vi "resetHomePosition.vi"(8 "error in (no error)":errorcluster, 11 "VISA Refnum in":refnum<visa-resource-name>) -> (0 "error out":errorcluster, 3 "VISA Refnum out":refnum<visa-resource-name>)   [LabVIEW 2014]
doc: "Newport Motion Controler\nThis VI reset HOME position\n\nAndré Romero - 2020\nandretec@ifsc.usp.br"
uses:
  <userlib>/Newport ESP301/Newport ESP301.lvlib
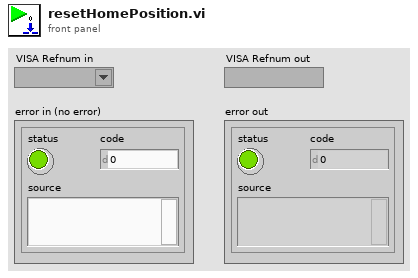
[diagram p1: front panel]
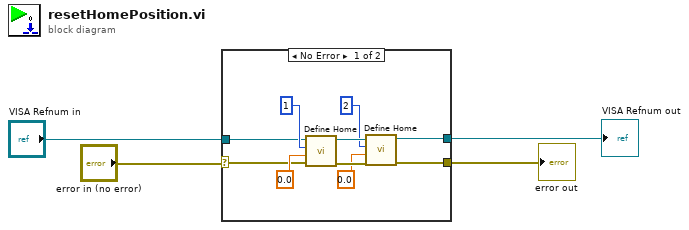
[diagram p0: block diagram]
diagram:
  n1 = case shown="No Error" "error in (no error)" {
    selector: "error in (no error)" -> [w5 w15]
    tunnel: [w8 w16] -> w4
    tunnel: [w7 w15] -> w3
    tunnel: "VISA Refnum in" -> [w6 w16]
    frame No Error {
      n2 = call <userlib>:"Define Home.vi"("error in (no error)"=w5, "Home Position (0 units)"=0.0, "Axis (1)"=1 ("y"), "VISA resource name"=w6) -> ("error out"=w13:errorcluster, "VISA resource name out"=w14:refnum<visa-resource-name>)  [unwired: 2 in]
      n3 = call <userlib>:"Define Home.vi"("error in (no error)"=w13, "Home Position (0 units)"=0.0, "Axis (1)"=2, "VISA resource name"=w14) -> ("error out"=w7:errorcluster, "VISA resource name out"=w8:refnum<visa-resource-name>)  [unwired: 2 in]
    }
    frame Error {
    }
  }
  "VISA Refnum out" <- w4
  "error out" <- w3
